vi "PID Autotuning Design.vi"   [LabVIEW 2017, in "NI_PID_autopid.lvlib"]
doc: "Implements autotuning using the tuning method associated with the polymorphic instance you select. This VI generates PID parameters based on the <B>Stimulus signal</B> and <B>Response signal</B> you specify. You can use this VI to generate initial parameters when you do not have sufficient information about the system you want to tune. You must manually select the polymorphic instance to use."
uses:
  <vilib>/addons/control/pid/NI_PID_autopid.lvlib
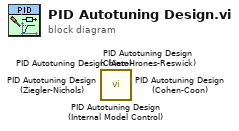
[diagram p0: block diagram]
diagram:
  n1 = call <vilib>:"PID Autotuning Design (Internal Model Control).vi"() -> ()  [unwired: 8 in, 4 out]
  n2 = call <vilib>:"PID Autotuning Design (Chien-Hrones-Reswick).vi"() -> ()  [unwired: 8 in, 4 out]
  n3 = call <vilib>:"PID Autotuning Design (Ziegler-Nichols).vi"() -> ()  [unwired: 8 in, 4 out]
  n4 = call <vilib>:"PID Autotuning Design (Cohen-Coon).vi"() -> ()  [unwired: 8 in, 4 out]
  n5 = call <vilib>:"PID Autotuning Design (Auto).vi"() -> ()  [unwired: 8 in, 4 out]
